vi "Numeric Field.vi"(8 "error in":errorcluster, 10 "Ctl Refnum":refnum<vi>, 11 "Column Name":string) -> (0 "error out":errorcluster, 3 "Field Configuration":refnum<class "Field Configuration.lvclass">)   [LabVIEW 2020, in "Basic Field Constructors.lvlib"]
uses:
  Basic Field Constructors.lvlib
  Basic Fields/Field Configurations/Field Configuration Class/Field Configuration.lvclass
  Database Libraries/Database Interfaces/Database data type.ctl
  <vilib>/Utility/Data Type/NI_Data Type.lvlib
  Database Libraries/Database Interfaces.lvlib
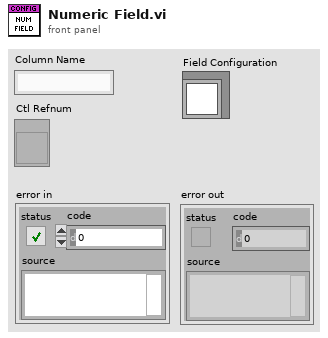
[diagram p1: front panel]
types:
  T1 = typedef "LVNumericRepresentation.ctl" = enum32{"Extended Precision", "Double Precision", "Single Precision", "Long", "Word", "Byte", "Unsigned Long", "Unsigned Word", "Unsigned Byte", "Complex Extended", "Complex Double", "Complex Single", "Quad", "Unsigned Quad", "Fixed-Point"}
  T2 = typedef "Database Interfaces.lvlib/Database data type.ctl" = enum16{"String", "Long (I32)", "Single (SGL)", "Double (DBL)", "Date/Time", "Binary"}
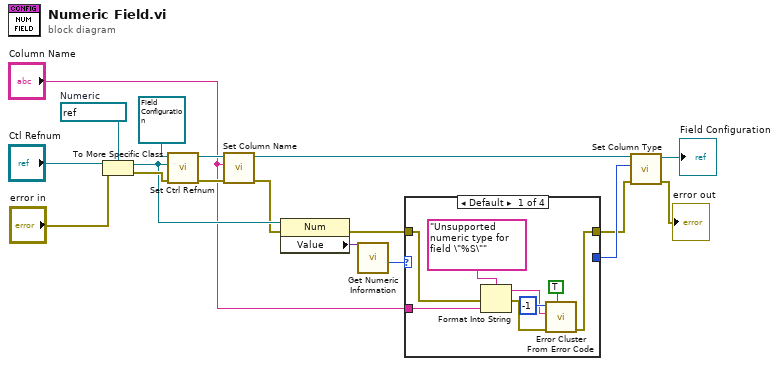
[diagram p0: block diagram]
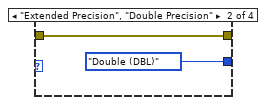
[diagram p2: hidden frame]
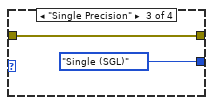
[diagram p3: hidden frame]
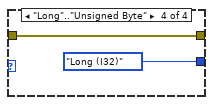
[diagram p4: hidden frame]
diagram:
  w13 = refnum<vi> refnum  # Numeric
  n1 = To More Specific Class(target class=w13, reference="Ctl Refnum", error in="error in") -> (specific class reference=w8:refnum<vi>, error out=w12:errorcluster)
  n2 = call-dynamic "Set Ctrl Refnum.vi"("error in (no error)"=w12, "Ctl Refnum"=w8, "Field Configuration in"=refnum<class "Field Configuration.lvclass"> refnum ("Basic Fields.lvlib:Field Configuration.lvclass")) -> ("error out"=w11:errorcluster, "Field Configuration out"=w17:refnum<class "Field Configuration.lvclass">)  [unwired: 7 in]
  n3 = call-dynamic "Set Column Name.vi"("error in (no error)"=w11, "Column Name"="Column Name", "Basic Column Configuration in"=w17) -> ("error out"=w5:errorcluster, "Basic Column Configuration out"=w16:refnum<class "Field Configuration.lvclass">)  [unwired: 7 in]
  n4 = property class="Num"(reference=w8, error in=w5) -> (error out=w4:errorcluster, "Value"=w7:variant)  [unwired: 1 out]
  n5 = call <vilib>:"Get Numeric Information.vi"("variant"=w7) -> ("representation"=w6:T1)  [unwired: 7 in, 3 out]
  n6 = case shown="Default" w6 {
    tunnel: w4 -> [w21 w27 w29 w31]
    tunnel: [_ Database_data_type."Double (DBL)" ("Column Type") Database_data_type."Single (SGL)" ("Column Type") Database_data_type."Long (I32)" ("Column Type")] -> w3
    tunnel: "Column Name" -> [w25 _ _ _]
    tunnel: [w19 w27 w29 w31] -> w1
    frame Default {
      n7 = Format Into String(format string="Unsupported numeric type for field \"%S\"", error in=w21, w25) -> (resulting string=w22:string, error out=w20:errorcluster)  [unwired: 1 in]
      n8 = call <vilib>:"Error Cluster From Error Code.vi"("show call chain? (False)"=TRUE, "error in (no error)"=w20, "error message (\"\")"=w22, "error code (0)"=-1) -> ("error out"=w19:errorcluster)  [unwired: 5 in]
    }
    frame "Extended Precision", "Double Precision" {
    }
    frame "Single Precision" {
    }
    frame "Long".."Unsigned Byte" {
    }
  }
  n9 = call-dynamic "Set Column Type.vi"("error in (no error)"=w1, "Column Type"=w3, "Basic Column Configuration in"=w16) -> ("error out"=→"error out":errorcluster, "Basic Column Configuration out"=→"Field Configuration":refnum<class "Field Configuration.lvclass">)  [unwired: 7 in]
